vi "svx_Colormap Get Run-time Shortcut Menu Label.vi"(11 "MenuRef":refnum<k9>) -> (1 "Disable item tags":string[](array[string])=["USER_SC_SCALE_LEGEND", "USER_SC_GRAPH_PALETTE", "USER_SC_CURSOR_LEGEND", "USER_SC_X_SCALE", "USER_SC_Y_SCALE", "USER_SC_Z_SCALE", "USER_SC_AUTOSCALE_X", "USER_SC_AUTOSCALE_Y", "USER_SC_AUTOSCALE_Z", "USER_SC_IGNORE_COLOR_ARRAY", "USER_SC_INTERPOLATE_COLOR", "USER_SC_SMOOTH_UPDATES", "USER_SC_LABEL", "USER_SC_CAPTION", "USER_SC_ORDER", "USER_SC_FREQ"], 2 "item tags":string[](array[string]), 3 "menu reference out":refnum<k9>)   [LabVIEW 2017, in "SVX Colormap.xctl"]
uses:
  <vilib>/addons/_XControls/Colormap/SVX Colormap.xctl
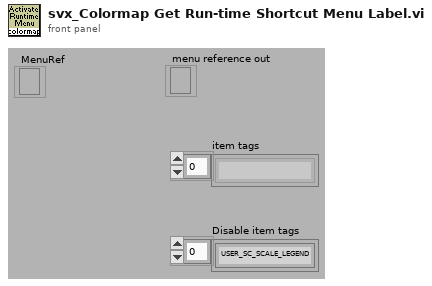
[diagram p1: front panel]
types:
  T1 = cluster{"menu tag":string, "item names":string, "item tags":string}[]
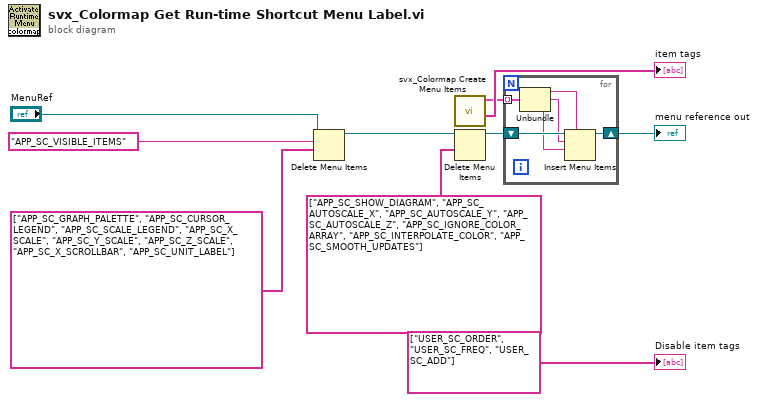
[diagram p0: block diagram]
diagram:
  n1 = Delete Menu Items(7:string[] ["APP_SC_GRAPH_PALETTE", "APP_SC_CURSOR_LEGEND", "APP_SC_SCALE_LEGEND", "APP_SC_X_SCALE", "APP_SC_Y_SCALE", "APP_SC_Z_SCALE", "APP_SC_X_SCROLLBAR", "APP_SC_UNIT_LABEL"] ("item tags"), 8:"APP_SC_VISIBLE_ITEMS", 9:"MenuRef") -> (3:w3:refnum<k9>)  [unwired: 1 in, 1 out]
  n2 = call <vilib>:"svx_Colormap Create Menu Items.vi"() -> ("item tags"=→"item tags":string[], "menu items"=w8:T1)  [unwired: 10 in]
  n3 = Delete Menu Items(7:string[] ["APP_SC_SHOW_DIAGRAM", "APP_SC_AUTOSCALE_X", "APP_SC_AUTOSCALE_Y", "APP_SC_AUTOSCALE_Z", "APP_SC_IGNORE_COLOR_ARRAY", "APP_SC_INTERPOLATE_COLOR", "APP_SC_SMOOTH_UPDATES"], 9:w3) -> (3:w7:refnum<k9>)  [unwired: 2 in, 1 out]
  n4 = for {
    shift-right: [w15] -> w10
    shift-left: w7 -> [w16]
    tunnel: w8 -> [w14] mode=indexing
    n5 = Unbundle(w14) -> ("menu tag"=w13:string, "item names"=w12:string, "item tags"=w11:string)
    n6 = Insert Menu Items(5:w13, 7:w11, 8:w12, 9:w16) -> (3:w15:refnum<k9>)  [unwired: 2 in, 2 out]
  }
  "menu reference out" <- w10
  "Disable item tags" <- string[] ["USER_SC_ORDER", "USER_SC_FREQ", "USER_SC_ADD"] ("Disable item tags")
